vi "Motor control with PID.vi"() -> ()   [LabVIEW 2013]
uses:
  <vilib>/eio/EIONode/EIONode.xnode
  <vilib>/rvi/eio/common/nirviEmuTemplateMethod_errors.vi
  <vilib>/addons/control/pid/fpga.llb/XNode/niFpgaPID.xnode
panel:
  in  "Update Insides Values":bool
  in  "Tab Control":enum32{"Motor 1", "Motor 2", "Motor 3"}(tab)
  in  "Position Reset":bool
  out "Speed Output":T1
  out "Position Output":T2
  in  "Velocity Interval (uSec)":i32
  in  "stop":bool
  in  "Control":T3={"Pulse Lenght DIO3"=10000, "Pulse Period 3"=20000, "Angle"=0}
  out "Inside values":T3
  in  "Encoder Intputs":T4={"Tach 1"="ConnectorB/DIO8", "Tach 2"="ConnectorB/DIO9"}
  in  "PID gains":T5={"proportional gain (Kc)"=1.0, "integral gain (Kc*Ts/Ti)"=1.66796875, "derivative gain (Kc*Td/Ts)"=0.0}
  in  "reset?":bool
  in  "Velocity wanted (Counts/Interval)":i16
  out "PID Output":i16
  out "Velocity (Counts/Interval)":i32
  out "Degree (absolute)":i32
  out "Degree (absolute) 2":i32
  out "Velocity (Counts/Interval) 2":i32
  out "PID Output 2":i16
  in  "Velocity wanted (Counts/Interval) 2":i16
  in  "reset? 2":bool
  in  "PID gains 2":T5={"proportional gain (Kc)"=1.0, "integral gain (Kc*Ts/Ti)"=1.66796875, "derivative gain (Kc*Td/Ts)"=0.0}
  in  "Encoder Intputs 2":T4={"Tach 1"="ConnectorB/DIO6", "Tach 2"="ConnectorB/DIO7"}
  out "Inside values 2":T3
  in  "Control 2":T3={"Pulse Lenght DIO3"=10000, "Pulse Period 3"=20000, "Angle"=0}
  in  "stop 2":bool
  in  "Velocity Interval (uSec) 2":i32
  out "Position Output 2":T2
  out "Speed Output 2":T1
  in  "Position Reset 2":bool
  in  "reset? 3":bool
  in  "PID gains 3":T5={"proportional gain (Kc)"=1.0, "integral gain (Kc*Ts/Ti)"=1.66796875, "derivative gain (Kc*Td/Ts)"=0.0}
  out "PID Output 3":i16
  in  "Velocity wanted (Counts/Interval) 3":i16
  in  "stop 3":bool
  in  "Control 3":T3={"Pulse Lenght DIO3"=10000, "Pulse Period 3"=20000, "Angle"=0}
  out "Inside values 3":T3
  in  "Position Reset 3":bool
  out "Degree (absolute) 3":i32
  out "Velocity (Counts/Interval) 3":i32
  out "Speed Output 3":T1
  out "Position Output 3":T2
  in  "Encoder Intputs 3":T4={"Tach 1"="ConnectorA/DIO8", "Tach 2"="ConnectorA/DIO9"}
  in  "Velocity Interval (uSec) 3":i32
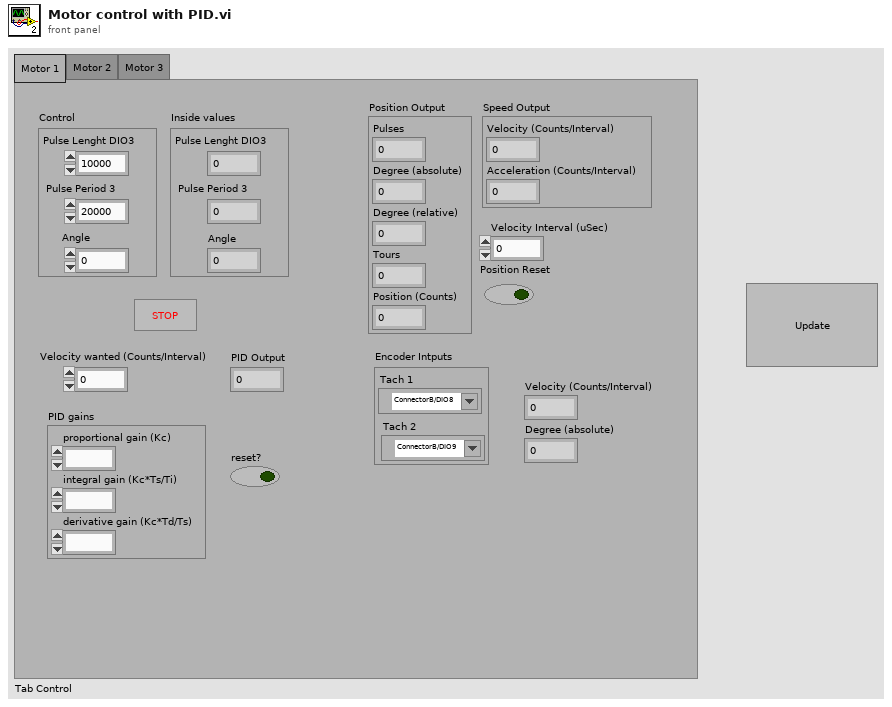
[diagram p1: front panel]
types:
  T1 = cluster{"Velocity (Counts/Interval)":i32, "Acceleration (Counts/Interval)":i32}
  T2 = cluster{"Pulses":i32, "Degree (absolute)":i32, "Degree (relative)":i32, "Tours":i32, "Position (Counts)":i32}
  T3 = cluster{"Pulse Lenght DIO3":i32, "Pulse Period 3":i32, "Angle":i32}
  T4 = cluster{"Tach 1":refnum<k21>, "Tach 2":refnum<k21>}
  T5 = cluster{"proportional gain (Kc)":fxp<+/-,16,8>, "integral gain (Kc*Ts/Ti)":fxp<+/-,16,8>, "derivative gain (Kc*Td/Ts)":fxp<+/-,16,8>}
  T6 = cluster{"Velocity Interval (uSec)":i32, "I/O Tach 1":bool, "I/O Tach 2":bool, "Position (Counts)":i16, "Boolean Variable 1":bool, "Tick Count(Ticks)":u32, "Position (Counts) 2":i16, "Acceleration (Counts/Interval)":i16, "Velocity (Counts/Interval":i16}
  T7 = cluster{"proportional gain (Kc)":i16, "integral gain (Kc*Ts/Ti)":i16, "derivative gain (Kc*Td/Ts)":i16}
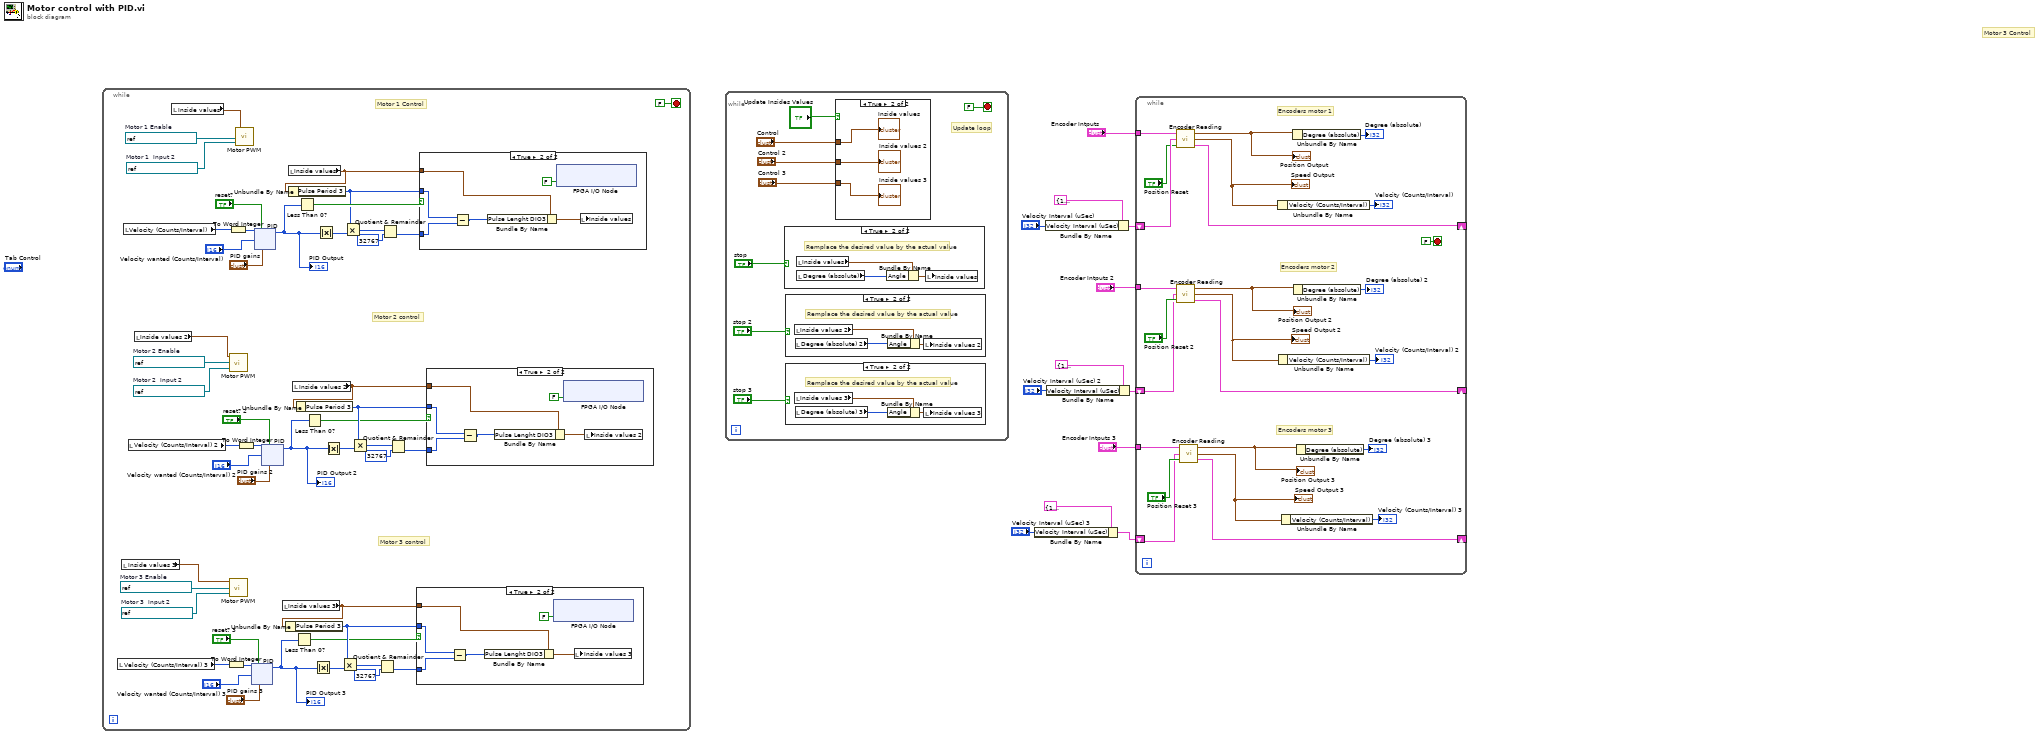
[diagram p0: block diagram]
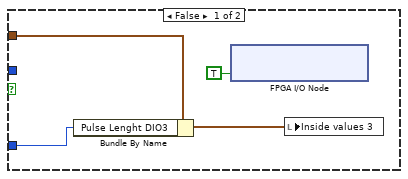
[diagram p2: hidden frame]
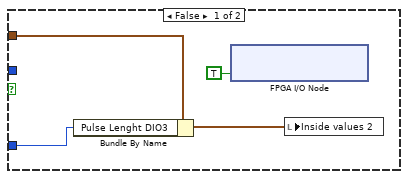
[diagram p3: hidden frame]
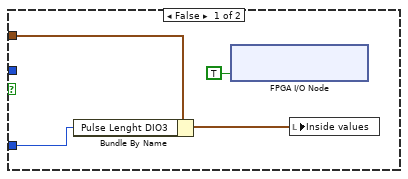
[diagram p4: hidden frame]
diagram:
  # "Motor 3 Control"
  n1 = while {
    stop <- FALSE stop-if-true
    w14 = refnum<k21> "ConnectorA/DIO0"  # Motor 3 Enable
    w13 = refnum<k21> "ConnectorA/DIO2"  # Motor 3  Input 2
    w17 = refnum<k21> "ConnectorB/DIO3"  # Motor 2 Enable
    w16 = refnum<k21> "ConnectorB/DIO5"  # Motor 2  Input 2
    w19 = refnum<k21> "ConnectorB/DIO0"  # Motor 1 Enable
    w20 = refnum<k21> "ConnectorB/DIO2"  # Motor 1  Input 2
    # "Motor 3 control"
    # "Motor 2 control"
    # "Motor 1 Control"
    n2 = local read "Velocity (Counts/Interval) 3"() -> (w27:i32)
    n3 = local read "Inside values 3"() -> (w15:T3)
    n4 = local read "Velocity (Counts/Interval)"() -> (w55:i32)
    n5 = local read "Velocity (Counts/Interval) 2"() -> (w40:i32)
    n6 = local read "Inside values 2"() -> (w18:T3)
    n7 = local read "Inside values"() -> (w21:T3)
    n8 = To Word Integer(number=w27) -> (16bit integer=w23:i16)
    n9 = call "Motor PWM.vi"("Motor Input 2"=w16, "Motor Enable"=w17, "Inside values"=w18) -> ()  [unwired: 1 in]
    n10 = call "Motor PWM.vi"("Motor Input 2"=w13, "Motor Enable"=w14, "Inside values"=w15) -> ()  [unwired: 1 in]
    n11 = To Word Integer(number=w55) -> (16bit integer=w60:i16)
    n12 = call "Motor PWM.vi"("Motor Input 2"=w20, "Motor Enable"=w19, "Inside values"=w21) -> ()  [unwired: 1 in]
    n13 = To Word Integer(number=w40) -> (16bit integer=w36:i16)
    n14 = xnode "PID"("process variable"=w23, "reset?"="reset? 3", "setpoint"="Velocity wanted (Counts/Interval) 3", "PID gains"="PID gains 3") -> ("output"=w31:i16)  [unwired: 1 in]
    "PID Output 3" <- w31
    n15 = xnode "PID"("process variable"=w60, "reset?"="reset?", "setpoint"="Velocity wanted (Counts/Interval)", "PID gains"="PID gains") -> ("output"=w51:i16)  [unwired: 1 in]
    "PID Output" <- w51
    n16 = xnode "PID"("process variable"=w36, "reset?"="reset? 2", "setpoint"="Velocity wanted (Counts/Interval) 2", "PID gains"="PID gains 2") -> ("output"=w44:i16)  [unwired: 1 in]
    "PID Output 2" <- w44
    n17 = local read "Inside values 3"() -> (w33:T3)
    n18 = Unbundle By Name(w33) -> ("Pulse Period 3"=w34:i32)
    n19 = local read "Inside values"() -> (w49:T3)
    n20 = Unbundle By Name(w49) -> ("Pulse Period 3"=w48:i32)
    n21 = local read "Inside values 2"() -> (w46:T3)
    n22 = Less Than 0?(x=w31) -> (x < 0?=w24:bool)
    n23 = Unbundle By Name(w46) -> ("Pulse Period 3"=w47:i32)
    n24 = Less Than 0?(x=w51) -> (x < 0?=w59:bool)
    n25 = Less Than 0?(x=w44) -> (x < 0?=w37:bool)
    n26 = Absolute Value(x=w31) -> (abs(x)=w29:i16)
    n27 = Absolute Value(x=w51) -> (abs(x)=w53:i16)
    n28 = Absolute Value(x=w44) -> (abs(x)=w42:i16)
    n29 = Multiply(x=w34, y=w29) -> (x*y=w30:i32)
    n30 = Multiply(x=w48, y=w53) -> (x*y=w52:i32)
    n31 = Multiply(x=w47, y=w42) -> (x*y=w43:i32)
    n32 = Quotient & Remainder(x=w30, y=i16 32767) -> (floor(x/y)=w32:i32)  [unwired: 1 out]
    n33 = Quotient & Remainder(x=w52, y=i16 32767) -> (floor(x/y)=w50:i32)  [unwired: 1 out]
    n34 = Quotient & Remainder(x=w43, y=i16 32767) -> (floor(x/y)=w45:i32)  [unwired: 1 out]
    n35 = case shown="True" w24 {
      tunnel: w32 -> [w63 w69]
      tunnel: w33 -> [w62 w66]
      tunnel: w34 -> [_ w70]
      frame False {
        n36 = Bundle By Name(cluster=w62, "Pulse Lenght DIO3"=w63) -> (w64:T3)
        n37 = xnode "FPGA I/O Node"("ConnectorB/DIO1"=TRUE ("ConnectorC/DIO7")) -> ()  [unwired: 1 in, 1 out]
        n38 = local write "Inside values 3"(w64) -> ()
      }
      frame True {
        n39 = Subtract(x=w70, y=w69) -> (x-y=w67:i32)
        n40 = Bundle By Name(cluster=w66, "Pulse Lenght DIO3"=w67) -> (w68:T3)
        n41 = xnode "FPGA I/O Node"("ConnectorA/DIO1"=FALSE ("ConnectorC/DIO7")) -> ()  [unwired: 1 in, 1 out]
        n42 = local write "Inside values 3"(w68) -> ()
      }
    }
    n43 = case shown="True" w59 {
      tunnel: w50 -> [w139 w145]
      tunnel: w49 -> [w138 w142]
      tunnel: w48 -> [_ w146]
      frame False {
        n44 = Bundle By Name(cluster=w138, "Pulse Lenght DIO3"=w139) -> (w140:T3)
        n45 = xnode "FPGA I/O Node"("ConnectorB/DIO1"=TRUE ("ConnectorC/DIO7")) -> ()  [unwired: 1 in, 1 out]
        n46 = local write "Inside values"(w140) -> ()
      }
      frame True {
        n47 = Subtract(x=w146, y=w145) -> (x-y=w143:i32)
        n48 = Bundle By Name(cluster=w142, "Pulse Lenght DIO3"=w143) -> (w144:T3)
        n49 = xnode "FPGA I/O Node"("ConnectorB/DIO1"=FALSE ("ConnectorC/DIO7")) -> ()  [unwired: 1 in, 1 out]
        n50 = local write "Inside values"(w144) -> ()
      }
    }
    n51 = case shown="True" w37 {
      tunnel: w45 -> [w101 w107]
      tunnel: w46 -> [w100 w104]
      tunnel: w47 -> [_ w108]
      frame False {
        n52 = Bundle By Name(cluster=w100, "Pulse Lenght DIO3"=w101) -> (w102:T3)
        n53 = xnode "FPGA I/O Node"("ConnectorB/DIO1"=TRUE ("ConnectorC/DIO7")) -> ()  [unwired: 1 in, 1 out]
        n54 = local write "Inside values 2"(w102) -> ()
      }
      frame True {
        n55 = Subtract(x=w108, y=w107) -> (x-y=w105:i32)
        n56 = Bundle By Name(cluster=w104, "Pulse Lenght DIO3"=w105) -> (w106:T3)
        n57 = xnode "FPGA I/O Node"("ConnectorB/DIO4"=FALSE ("ConnectorC/DIO7")) -> ()  [unwired: 1 in, 1 out]
        n58 = local write "Inside values 2"(w106) -> ()
      }
    }
  }
  n59 = while {
    stop <- FALSE stop-if-true
    # "Update loop"
    n60 = case shown="True" "stop" {
      frame False {
      }
      frame True {
        # "Remplace the desired value by the actual value"
        n61 = local read "Inside values"() -> (w192:T3)
        n62 = local read "Degree (absolute)"() -> (w191:i32)
        n63 = Bundle By Name(cluster=w192, "Angle"=w191) -> (w190:T3)
        n64 = local write "Inside values"(w190) -> ()
      }
    }
    n65 = case shown="True" "stop 2" {
      frame False {
      }
      frame True {
        # "Remplace the desired value by the actual value"
        n66 = local read "Inside values 2"() -> (w189:T3)
        n67 = local read "Degree (absolute) 2"() -> (w188:i32)
        n68 = Bundle By Name(cluster=w189, "Angle"=w188) -> (w187:T3)
        n69 = local write "Inside values 2"(w187) -> ()
      }
    }
    n70 = case shown="True" "stop 3" {
      frame False {
      }
      frame True {
        # "Remplace the desired value by the actual value"
        n71 = local read "Inside values 3"() -> (w186:T3)
        n72 = local read "Degree (absolute) 3"() -> (w185:i32)
        n73 = Bundle By Name(cluster=w186, "Angle"=w185) -> (w184:T3)
        n74 = local write "Inside values 3"(w184) -> ()
      }
    }
    n75 = case shown="True" "Update Insides Values" {
      tunnel: "Control" -> [_ w195]
      tunnel: "Control 2" -> [_ w194]
      tunnel: "Control 3" -> [_ w193]
      frame False {
      }
      frame True {
        "Inside values" <- w195
        "Inside values 2" <- w194
        "Inside values 3" <- w193
      }
    }
  }
  n76 = Bundle By Name(cluster=T6 {"Velocity Interval (uSec)"=1000000, "I/O Tach 1"=FALSE, "I/O Tach 2"=FALSE, "Position (Counts)"=0, "Boolean Variable 1"=FALSE, "Tick Count(Ticks)"=0, "Position (Counts) 2"=0, "Acceleration (Counts/Interval)"=0, "Velocity (Counts/Interval"=0} ("Values"), "Velocity Interval (uSec)"="Velocity Interval (uSec) 3") -> (w2:T6)
  n77 = Bundle By Name(cluster=T6 {"Velocity Interval (uSec)"=1000000, "I/O Tach 1"=FALSE, "I/O Tach 2"=FALSE, "Position (Counts)"=0, "Boolean Variable 1"=FALSE, "Tick Count(Ticks)"=0, "Position (Counts) 2"=0, "Acceleration (Counts/Interval)"=0, "Velocity (Counts/Interval"=0} ("Values"), "Velocity Interval (uSec)"="Velocity Interval (uSec)") -> (w9:T6)
  n78 = Bundle By Name(cluster=T6 {"Velocity Interval (uSec)"=1000000, "I/O Tach 1"=FALSE, "I/O Tach 2"=FALSE, "Position (Counts)"=0, "Boolean Variable 1"=FALSE, "Tick Count(Ticks)"=0, "Position (Counts) 2"=0, "Acceleration (Counts/Interval)"=0, "Velocity (Counts/Interval"=0} ("Values"), "Velocity Interval (uSec)"="Velocity Interval (uSec) 2") -> (w4:T6)
  n79 = while {
    shift-right: [w217] -> _
    shift-left: w9 -> [w218]
    tunnel: "Encoder Intputs" -> [w219]
    shift-right: [w205] -> _
    shift-left: w4 -> [w206]
    tunnel: "Encoder Intputs 2" -> [w204]
    shift-right: [w196] -> _
    shift-left: w2 -> [w198]
    tunnel: "Encoder Intputs 3" -> [w197]
    stop <- FALSE stop-if-true
    # "Encoders motor 3"
    # "Encoders motor 2"
    # "Encoders motor 1"
    n80 = call "Encoder Reading.vi"("Position Reset"="Position Reset", "Values"=w218, "Encoder Intputs"=w219) -> ("output cluster"=w217:T6, "Speed Output"=w213:T1, "Position Output"=w214:T2)
    "Position Output" <- w214
    "Speed Output" <- w213
    n81 = call "Encoder Reading.vi"("Position Reset"="Position Reset 2", "Values"=w206, "Encoder Intputs"=w204) -> ("output cluster"=w205:T6, "Speed Output"=w210:T1, "Position Output"=w209:T2)
    "Position Output 2" <- w209
    "Speed Output 2" <- w210
    n82 = call "Encoder Reading.vi"("Position Reset"="Position Reset 3", "Values"=w198, "Encoder Intputs"=w197) -> ("output cluster"=w196:T6, "Speed Output"=w202:T1, "Position Output"=w201:T2)
    "Position Output 3" <- w201
    "Speed Output 3" <- w202
    n83 = Unbundle By Name(w213) -> ("Velocity (Counts/Interval)"=→"Velocity (Counts/Interval)":i32)
    n84 = Unbundle By Name(w210) -> ("Velocity (Counts/Interval)"=→"Velocity (Counts/Interval) 2":i32)
    n85 = Unbundle By Name(w202) -> ("Velocity (Counts/Interval)"=→"Velocity (Counts/Interval) 3":i32)
    n86 = Unbundle By Name(w214) -> ("Degree (absolute)"=→"Degree (absolute)":i32)
    n87 = Unbundle By Name(w209) -> ("Degree (absolute)"=→"Degree (absolute) 2":i32)
    n88 = Unbundle By Name(w201) -> ("Degree (absolute)"=→"Degree (absolute) 3":i32)
  }
